vi "Digital Output Engine.vi"(5 "Main Engine Q":refnum<queue>, 7 "TCP Enigine Q":refnum<queue>, 8 "error in (no error)":errorcluster, 10 "Engine Name":string, 11 "Varient Data":variant) -> (0 "error out":errorcluster)   [LabVIEW 2024]
doc: "All Rights Reserved © 2017 SyncSols"
uses:
  Controls/Digital Output State Machine Data Cluster.ctl
  TCP Engine/Controls/TCP Engine I&O  Interupt Cluster.ctl
  Controls/DIO Configuration cluster.ctl
  Controls/DIO Interface Data.ctl
  SubVIs/Digital Dynamic Cluster.ctl
  Controls/DIO Commad Q Cluster.ctl
  Main Engine/Controls/Main Engine JSON Command State.ctl
  Host-DQMH/Configuration/DO Channel's.ctl
  Controls/Digital Output SMCases.ctl
  Main Engine/Controls/Main Engine Engine No.Options.ctl
  Host-DQMH/Configuration/All Interface Data.ctl
  Host-DQMH/Configuration/Analog Input Single Channel Data--Cluster.ctl
  Host-DQMH/Configuration/Config-Channel Type.ctl
  Host-DQMH/Configuration/Channel Sub-Type.ctl
  Analog Output/Controls/AO Timing Cluster.ctl
  Main Engine/Controls/Main Engine Config Confirmation Cluster.ctl
  <vilib>/DAQmx/create/channels.llb/DAQmx Create Channel (DO-Digital Output).vi
  TCP Engine/TCP Engine.lvlib
  Host-DQMH/Configuration/Configuration.lvlib
panel:
  out "Array":string[](array[string])
  in  "Data Cluster":T1={"Array"=[], "Boolean"=FALSE, "Engine Name"="", "Main Engine Response Q"=refnum, "TCP Engine Response Q"=refnum, "Varient Data"=variant(string ""), "Interupt Q"=refnum, "Start Notifier"=refnum, "Stop Notifier"=refnum, "DIO Configuration Cluster"={"Interface"="", "Interface Data"={"Command"="", "SubCmd"="", "Frequency"=0, "Data"=[]}}, "DO Task"="", "Command Q"=refnum, "DO Config Data"=[], "Log File Path"=path ""}
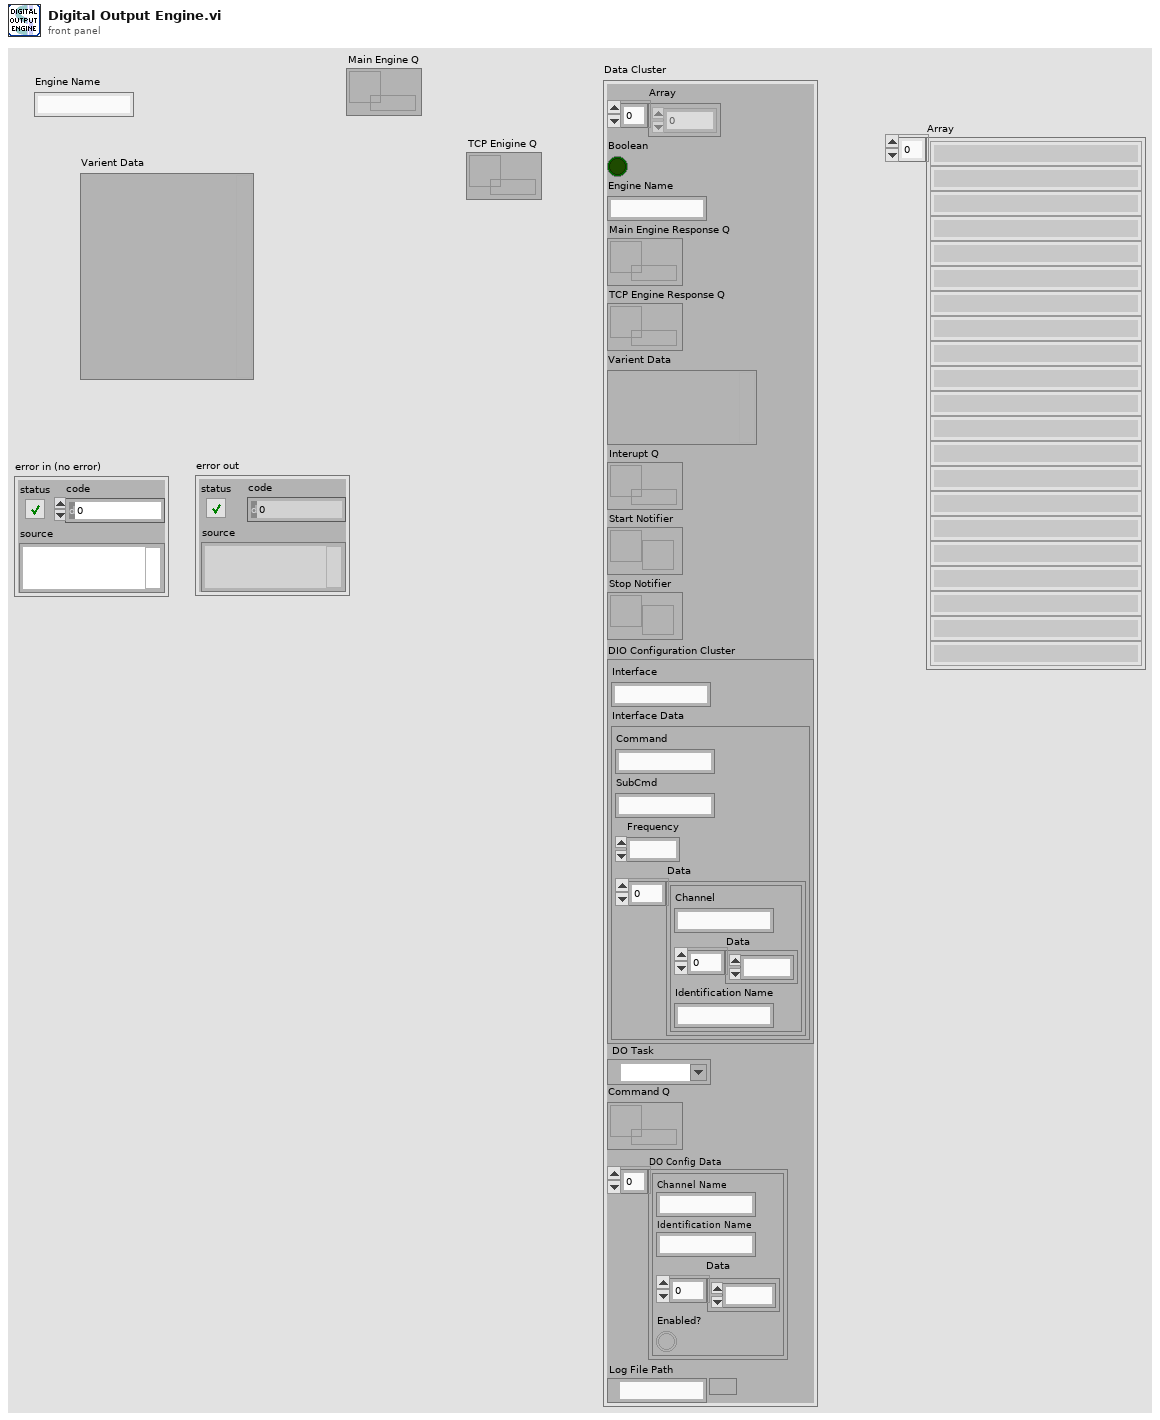
[diagram p1: front panel]
types:
  T1 = typedef "Digital Output State Machine Data Cluster.ctl" = cluster{"Array":dbl[], "Boolean":bool, "Engine Name":string, "Main Engine Response Q":refnum<queue>, "TCP Engine Response Q":refnum<queue>, "Varient Data":variant, "Interupt Q":refnum<queue>, "Start Notifier":refnum<notifier>, "Stop Notifier":refnum<notifier>, "DIO Configuration Cluster":T2, "DO Task":refnum<k21>, "Command Q":refnum<queue>, "DO Config Data":T5, "Log File Path":path}
  T2 = typedef "DIO Configuration cluster.ctl" = cluster{"Interface":string, "Interface Data":T3}
  T3 = typedef "DIO Interface Data.ctl" = cluster{"Command":string, "SubCmd":string, "Frequency":u16, "Data":T4[]}
  T4 = typedef "Digital Dynamic Cluster.ctl" = cluster{"Channel":string, "Data":u8[], "Identification Name":string}
  T5 = typedef "Configuration.lvlib/DO Channel's.ctl" = cluster{"Channel Name":string, "Identification Name":string, "Data":u8[], "Enabled?":bool}[]
  T6 = typedef "Digital Output SMCases.ctl" = enum16{">Poll", ".........State Machine.........", ">Init", ">Error", ">Exit", "..........Digital Output Engine Case..........", ">JSON to LVDATA", ">Gen Dyn Data", ">Get Command", ">Configure", ">Start", ">Generate", ">Stop"}
  T7 = typedef "DIO Commad Q Cluster.ctl" = cluster{"Interface":string, "Interface Data":cluster{"Command":string, "SubCmd":string, "Frequency":u16, "Data":T4[]}, "Command State":T8}
  T8 = typedef "Main Engine JSON Command State.ctl" = enum16{"Configure", "Start", "Exit"}
  T9 = typedef "TCP Engine.lvlib/TCP Engine I&O  Interupt Cluster.ctl" = cluster{" Stop":bool, "JSON Variant":variant}
  T10 = typedef "Main Engine Engine No.Options.ctl" = enum16{"Init", "Update", "Response", "Get"}
  T11 = typedef "Configuration.lvlib/All Interface Data.ctl" = cluster{"DI Config Data":T5, "DO Config Data":T5, "AI Config Data's":cluster{"Module Name":string, "AI Channel's Data":T12[], "Analog Input Timing":T15}[]}
  T12 = typedef "Configuration.lvlib/Analog Input Single Channel Data--Cluster.ctl" = cluster{"Channel Name":string, "Identification Name":string, "Channel Type":T13, "Sub-Type":T14, "Data":string, "Enabled?":bool}
  T13 = typedef "Configuration.lvlib/Config-Channel Type.ctl" = enum16{"Voltage", "Current", "Thermocouple", "Acclerometer"}
  T14 = typedef "Configuration.lvlib/Channel Sub-Type.ctl" = enum16{"None", "Pressure", "Force"}
  T15 = typedef "AO Timing Cluster.ctl" = cluster{"samples per channel":i32, "sample mode":i32, "Sampling Rate":dbl}
  T16 = typedef "Main Engine Config Confirmation Cluster.ctl" = cluster{"Command":string, "Interface":string, "Status":string, "Board":string}
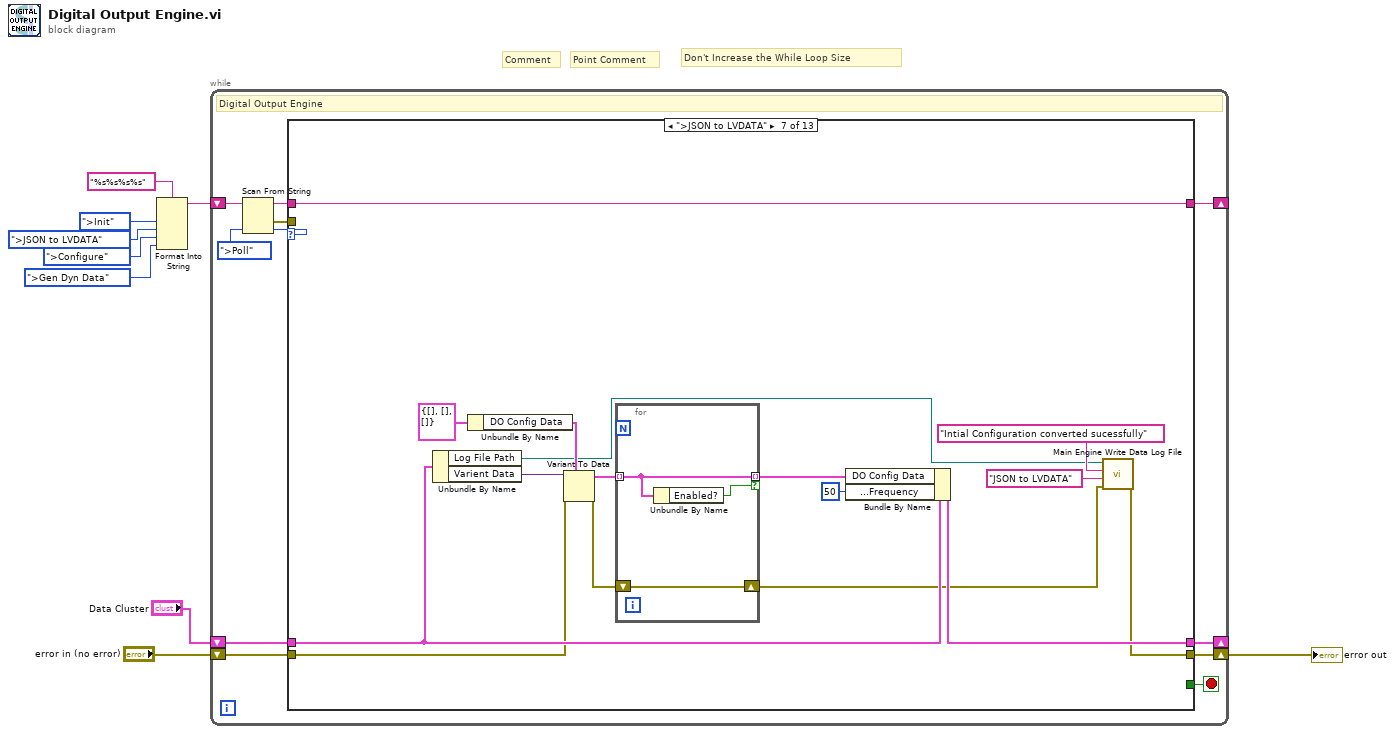
[diagram p0: block diagram]
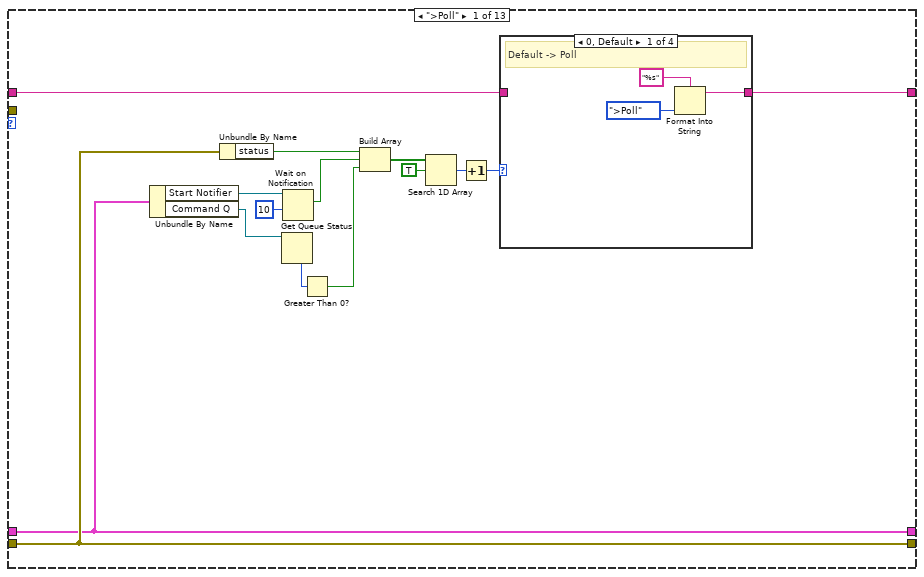
[diagram p2: hidden frame]
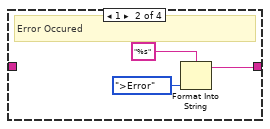
[diagram p3: hidden frame]
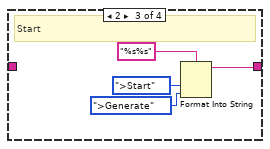
[diagram p4: hidden frame]
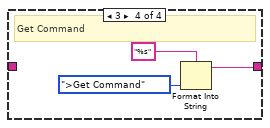
[diagram p5: hidden frame]
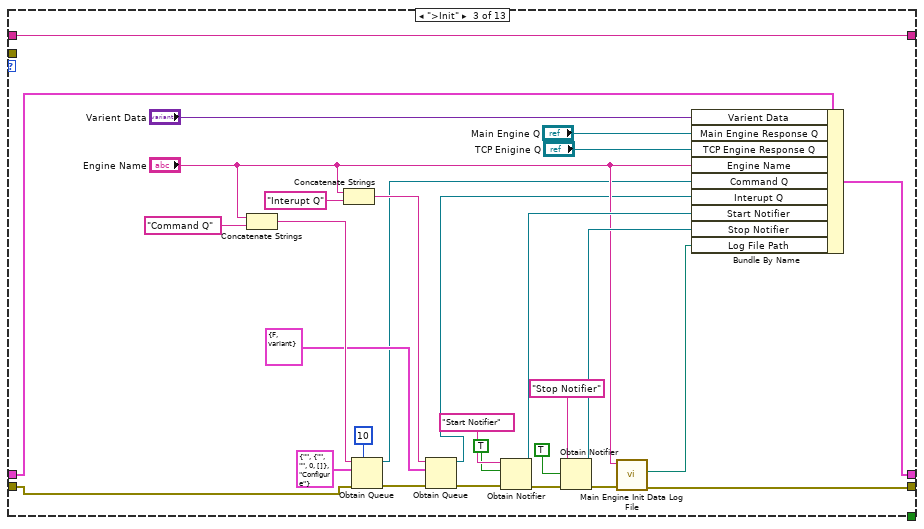
[diagram p7: hidden frame]
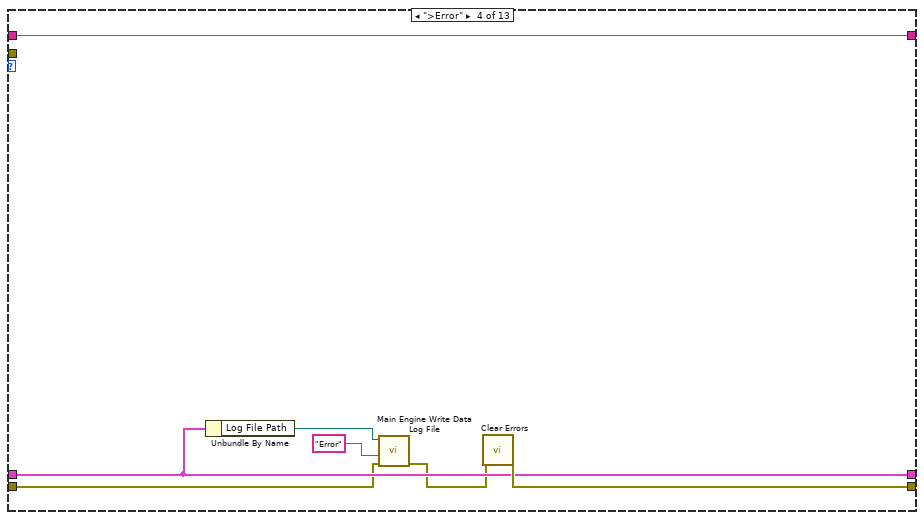
[diagram p8: hidden frame]
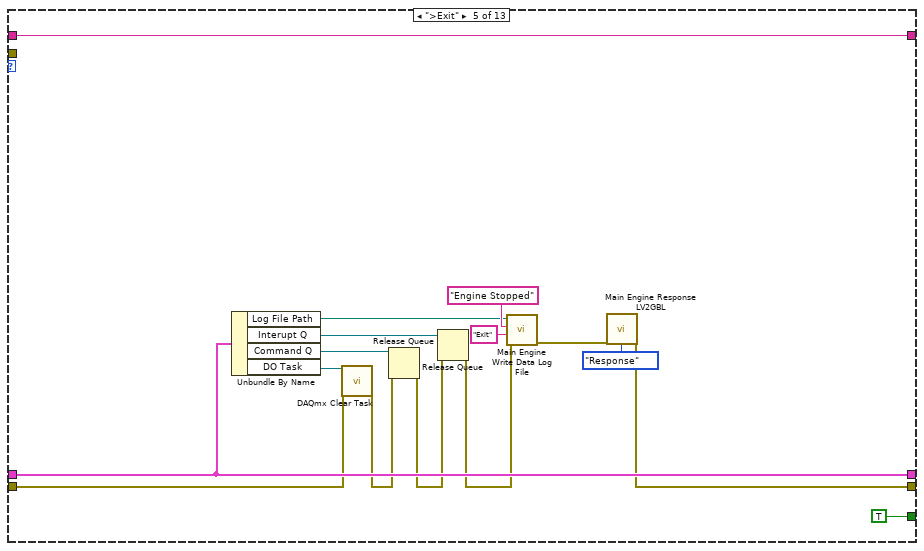
[diagram p9: hidden frame]
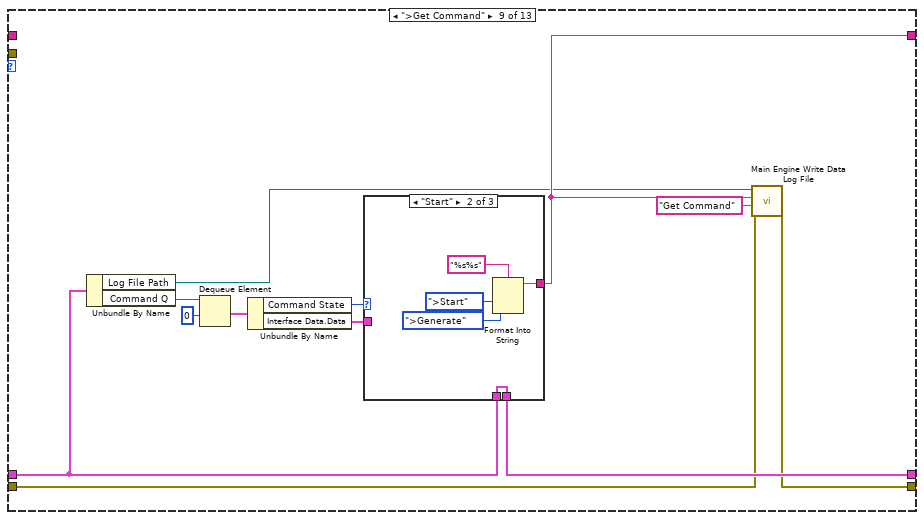
[diagram p12: hidden frame]
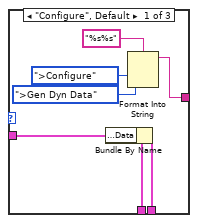
[diagram p13: hidden frame]
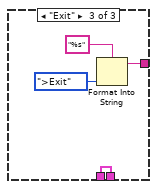
[diagram p14: hidden frame]
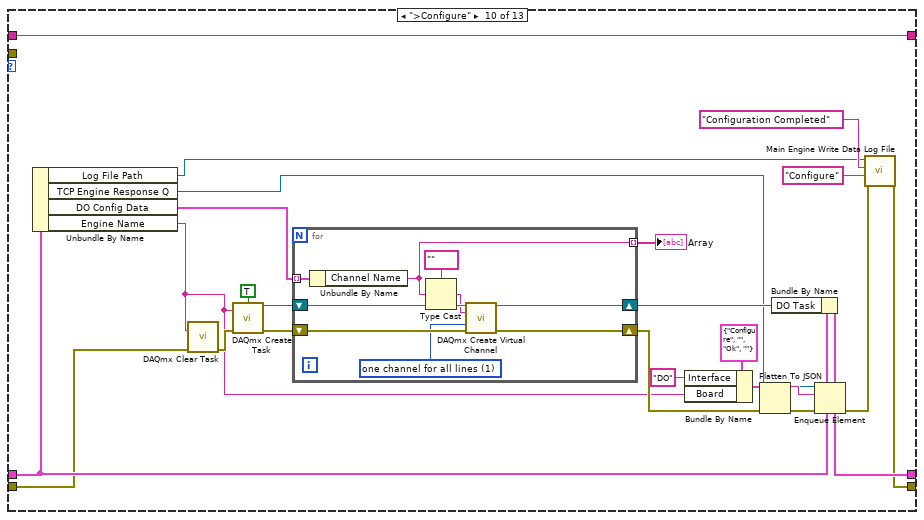
[diagram p15: hidden frame]
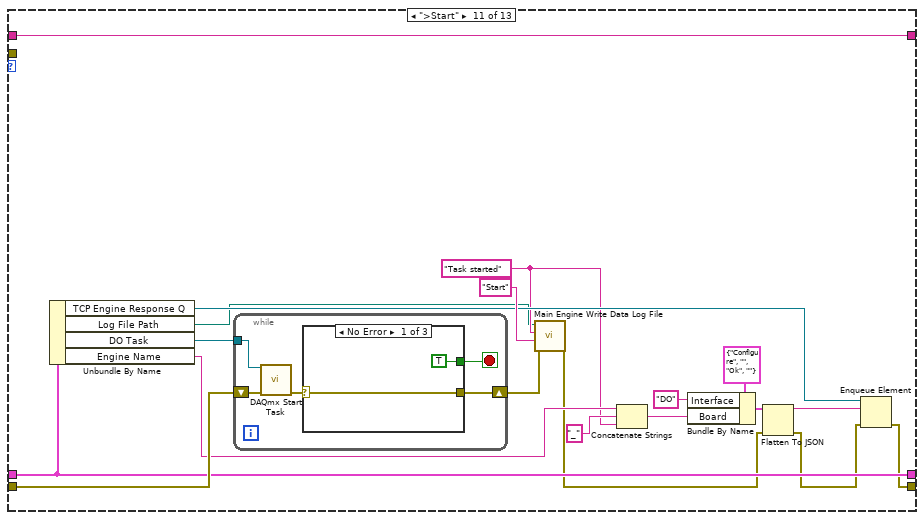
[diagram p16: hidden frame]
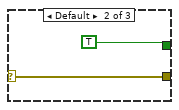
[diagram p17: hidden frame]
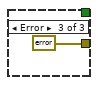
[diagram p18: hidden frame]
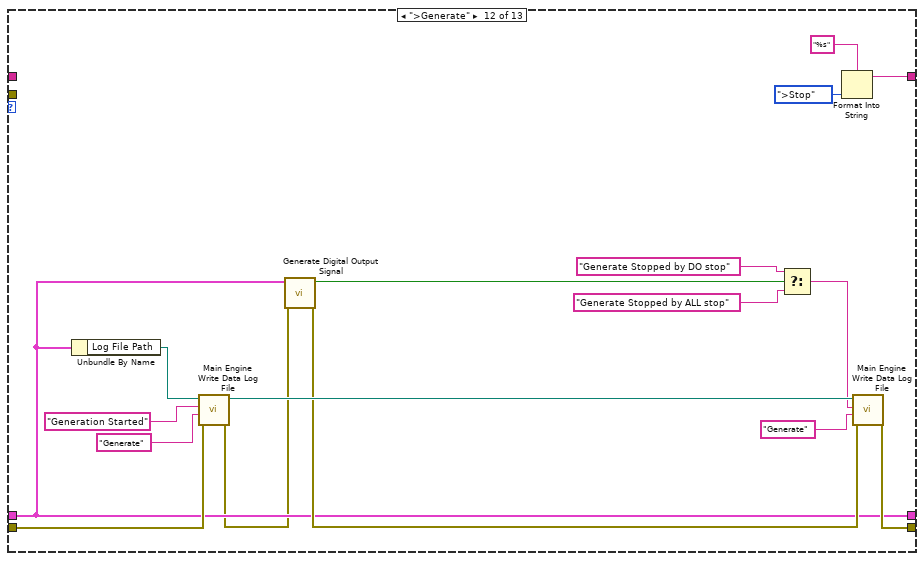
[diagram p19: hidden frame]
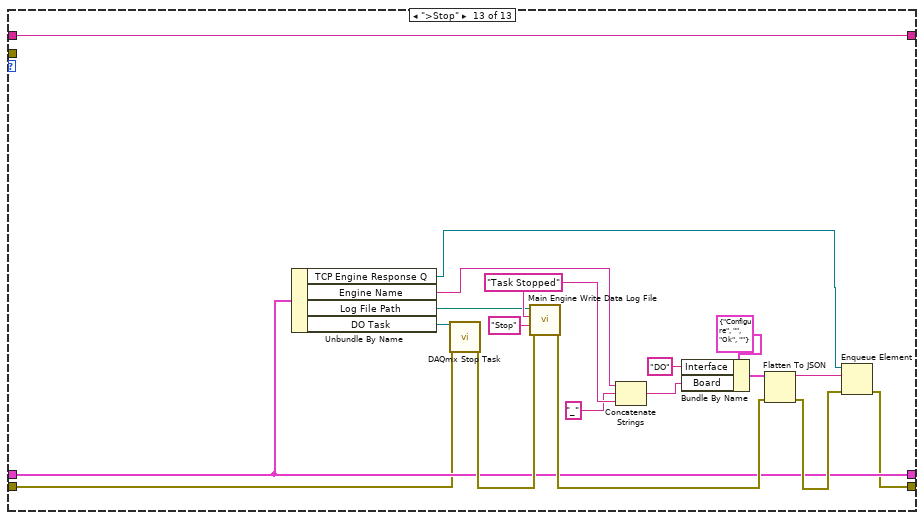
[diagram p20: hidden frame]
diagram:
  # "Don't Increase the While Loop Size"
  # "Point Comment"
  # "Comment"
  n1 = Format Into String(format string="%s%s%s%s", Digital_Output_SMCases.">Init" ("SM Cases Options"), Digital_Output_SMCases.">JSON to LVDATA" ("input 2"), Digital_Output_SMCases.">Configure" ("input 3"), Digital_Output_SMCases.">Gen Dyn Data" ("input 3")) -> (resulting string=w8:string)  [unwired: 2 in, 1 out]
  n2 = while {
    shift-right: [w15] -> _
    shift-left: w8 -> [w20]
    shift-right: [w13] -> w5
    shift-left: "error in (no error)" -> [w14]
    shift-right: [w11] -> _
    shift-left: "Data Cluster" -> [w10]
    stop <- w12 stop-if-true
    # "Digital Output Engine"
    n3 = Scan From String(input string=w20, default 1=Digital_Output_SMCases.">Poll" ("SM Cases Options")) -> (remaining string=w16:string, error out=w18:errorcluster, output 1=w17:T6)  [unwired: 3 in, 1 out]
    n4 = case shown="\">JSON to LVDATA\"" w17 {
      tunnel: w18 -> [_ _ _ _ _ _ _ _ _ _ _ _ _]
      tunnel: w16 -> [w35 w51 w80 w87 w103 w106 w122 w128 _ w180 w208 _ w254]
      tunnel: [w34 w51 w80 w87 w103 w106 w122 w128 w131 w180 w208 w229 w254] -> w15
      tunnel: w14 -> [w33 w50 w60 w83 w92 w105 w115 w126 w132 w176 w207 w235 w238]
      tunnel: [w33 w50 w61 w86 w90 w105 w119 w126 w133 w172 w191 w231 w237] -> w13
      tunnel: [_ _ _ _ TRUE _ _ _ _ _ _ _ _] -> w12
      tunnel: [w27 w49 w79 w84 w101 w104 w120 w127 w135 w174 w206 w221 w239] -> w11
      tunnel: w10 -> [w27 w49 w53 w84 w101 w104 w121 w127 w134 w179 w206 w221 w239]
      frame ">Poll" {
        n5 = Unbundle By Name(w27) -> ("Start Notifier"=w26:refnum<notifier>, "Command Q"=w24:refnum<queue>)
        n6 = Unbundle By Name(w33) -> ("status"=w32:bool)
        n7 = Get Queue Status(queue=w24) -> (# elements in queue=w23:i32)  [unwired: 2 in, 7 out]
        n8 = Wait on Notification(notifier=w26, timeout in ms (-1)=10) -> (notification=w25:bool)  [unwired: 2 in, 3 out]
        n9 = Greater Than 0?(x=w23) -> (x > 0?=w22:bool)
        n10 = Build Array(w32, w25, w22) -> (w31:bool[])
        n11 = Search 1D Array(1D array=w31, element=TRUE) -> (index of element=w29:i32)  [unwired: 1 in]
        n12 = Increment(x=w29) -> (x+1=w28:i32)
        n13 = case shown="0, Default" w28 {
          tunnel: w35 -> [_ _ _ _]
          tunnel: [w36 w39 w43 w46] -> w34
          frame 0, Default {
            # "Default -> Poll"
            n14 = Format Into String(format string="%s", Digital_Output_SMCases.">Poll" ("SM Cases Options")) -> (resulting string=w36:string)  [unwired: 2 in, 1 out]
          }
          frame 1 {
            # "Error Occured"
            n15 = Format Into String(format string="%s", Digital_Output_SMCases.">Error" ("SM Cases Options")) -> (resulting string=w39:string)  [unwired: 2 in, 1 out]
          }
          frame 2 {
            # "Start"
            n16 = Format Into String(format string="%s%s", Digital_Output_SMCases.">Start" ("SM Cases Options"), Digital_Output_SMCases.">Generate" ("input 2")) -> (resulting string=w43:string)  [unwired: 2 in, 1 out]
          }
          frame 3 {
            # "Get Command"
            n17 = Format Into String(format string="%s", Digital_Output_SMCases.">Get Command" ("SM Cases Options")) -> (resulting string=w46:string)  [unwired: 2 in, 1 out]
          }
        }
      }
      frame ".........State Machine........." {
      }
      frame ">Init" {
        n18 = Concatenate Strings("Engine Name", "Command Q" ("string")) -> (w76:string)
        n19 = Concatenate Strings("Engine Name", "Interupt Q" ("string")) -> (w73:string)
        n20 = Obtain Queue(max queue size (-1, unlimited)=10, name (unnamed)=w76, element data type=T7 {"Interface"="", "Interface Data"={"Command"="", "SubCmd"="", "Frequency"=0, "Data"=[]}, "Command State"=enum."Configure"} ("DIO Command Q Cluster"), error in (no error)=w60) -> (queue out=w58:refnum<queue>, error out=w78:errorcluster)  [unwired: 1 in, 1 out]
        n21 = Obtain Queue(name (unnamed)=w73, element data type=T9 {" Stop"=FALSE, "JSON Variant"=variant(string "")} ("I/O  Interupt Cluster"), error in (no error)=w78) -> (queue out=w56:refnum<queue>, error out=w66:errorcluster)  [unwired: 2 in, 1 out]
        n22 = Obtain Notifier(name (unnamed)="Start Notifier", notification data type=TRUE, error in (no error)=w66) -> (notifier out=w64:refnum<notifier>, error out=w71:errorcluster)  [unwired: 1 in, 1 out]
        n23 = Obtain Notifier(name (unnamed)="Stop Notifier", notification data type=TRUE, error in (no error)=w71) -> (notifier out=w63:refnum<notifier>, error out=w67:errorcluster)  [unwired: 1 in, 1 out]
        n24 = call "Main Engine Init Data Log File.vi"("error in"=w67, "Engine Name"="Engine Name") -> ("error out"=w61:errorcluster, "Log File Path"=w52:path)  [unwired: 8 in]
        n25 = Bundle By Name(cluster=w53, "Varient Data"="Varient Data", "Main Engine Response Q"="Main Engine Q", "TCP Engine Response Q"="TCP Enigine Q", "Engine Name"="Engine Name", "Command Q"=w58, "Interupt Q"=w56, "Start Notifier"=w64, "Stop Notifier"=w63, "Log File Path"=w52) -> (w79:T1)
      }
      frame ">Error" {
        n26 = Unbundle By Name(w84) -> ("Log File Path"=w81:path)
        n27 = call "Main Engine Write Data Log File.vi"("error in"=w83, "State"="Error" ("Input Data"), "Log file path In"=w81) -> ("error out"=w82:errorcluster)  [unwired: 7 in, 1 out]
        n28 = call <vilib>:"Clear Errors.vi"("error in (no error)"=w82) -> ("error out"=w86:errorcluster)  [unwired: 5 in, 1 out]
      }
      frame ">Exit" {
        n29 = Unbundle By Name(w101) -> ("Log File Path"=w88:path, "Interupt Q"=w99:refnum<queue>, "Command Q"=w100:refnum<queue>, "DO Task"=w91:refnum<k21>)
        n30 = call <vilib>:"DAQmx Clear Task.vi"("task in"=w91, "error in"=w92) -> ("error out"=w93:errorcluster)  [unwired: 13 in]
        n31 = Release Queue(queue=w100, error in (no error)=w93) -> (error out=w98:errorcluster)  [unwired: 1 in, 2 out]
        n32 = Release Queue(queue=w99, error in (no error)=w98) -> (error out=w97:errorcluster)  [unwired: 1 in, 2 out]
        n33 = call "Main Engine Write Data Log File.vi"("error in"=w97, "State"="Exit", "Input Data"="Engine Stopped", "Log file path In"=w88) -> ("error out"=w96:errorcluster)  [unwired: 6 in, 1 out]
        n34 = call "Main Engine Response LV2GBL.vi"("Options"=Main_Engine_Engine_No.Options."Response", "error in"=w96) -> ("error out"=w90:errorcluster)  [unwired: 7 in, 2 out]
      }
      frame "..........Digital Output Engine Case.........." {
      }
      frame ">JSON to LVDATA" {
        n35 = Unbundle By Name(w121) -> ("Log File Path"=w107:path, "Varient Data"=w116:variant)
        n36 = Unbundle By Name(T11 {"DI Config Data"=[], "DO Config Data"=[], "AI Config Data's"=[]} ("Interface Data")) -> ("DO Config Data"=w113:T5)
        n37 = Variant To Data(error in=w115, type=w113, Variant=w116) -> (data=w111:T5, error out=w109:errorcluster)
        n38 = for {
          tunnel: w111 -> [w125] mode=indexing
          tunnel: [w125] -> w110 mode=indexing if=w124
          shift-right: [w123] -> w108
          shift-left: w109 -> [w123]
          n39 = Unbundle By Name(w125) -> ("Enabled?"=w124:bool)
        }
        n40 = Bundle By Name(cluster=w121, "DO Config Data"=w110, "DIO Configuration Cluster.Interface Data.Frequency"=u16 50) -> (w120:T1)
        n41 = call "Main Engine Write Data Log File.vi"("error in"=w108, "State"="JSON to LVDATA", "Input Data"="Intial Configuration converted sucessfully", "Log file path In"=w107) -> ("error out"=w119:errorcluster)  [unwired: 6 in, 1 out]
      }
      frame ">Gen Dyn Data" {
      }
      frame ">Get Command" {
        n42 = Unbundle By Name(w134) -> ("Log File Path"=w129:path, "Command Q"=w140:refnum<queue>)
        n43 = Dequeue Element(queue=w140, timeout in ms (-1)=0) -> (element=w138:T7)  [unwired: 1 in, 3 out]
        n44 = Unbundle By Name(w138) -> ("Command State"=w137:T8, "Interface Data.Data"=w136:T4[])
        n45 = case shown="\"Start\"" w137 {
          tunnel: w134 -> [w147 w152 w156]
          tunnel: w136 -> [w146 _ _]
          tunnel: [w145 w152 w156] -> w135
          tunnel: [w142 w148 w153] -> w131
          frame "Configure", Default {
            n46 = Bundle By Name(cluster=w147, "DIO Configuration Cluster.Interface Data.Data"=w146) -> (w145:T1)
            n47 = Format Into String(format string="%s%s", Digital_Output_SMCases.">Configure" ("input 1"), Digital_Output_SMCases.">Gen Dyn Data" ("input 1")) -> (resulting string=w142:string)  [unwired: 2 in, 1 out]
          }
          frame "Start" {
            n48 = Format Into String(format string="%s%s", Digital_Output_SMCases.">Start" ("input 1"), Digital_Output_SMCases.">Generate" ("input 2")) -> (resulting string=w148:string)  [unwired: 2 in, 1 out]
          }
          frame "Exit" {
            n49 = Format Into String(format string="%s", Digital_Output_SMCases.">Exit" ("input 1")) -> (resulting string=w153:string)  [unwired: 2 in, 1 out]
          }
        }
        n50 = call "Main Engine Write Data Log File.vi"("error in"=w132, "State"="Get Command", "Input Data"=w131, "Log file path In"=w129) -> ("error out"=w133:errorcluster)  [unwired: 6 in, 1 out]
      }
      frame ">Configure" {
        n51 = Unbundle By Name(w179) -> ("Log File Path"=w157:path, "TCP Engine Response Q"=w165:refnum<queue>, "DO Config Data"=w159:T5, "Engine Name"=w161:string)
        n52 = call <vilib>:"DAQmx Clear Task.vi"("task in"=w161, "error in"=w176) -> ("error out"=w177:errorcluster)  [unwired: 13 in]
        n53 = call <vilib>:"DAQmx Create Task.vi"("new task name"=w161, "auto cleanup"=TRUE, "error in"=w177) -> ("task out"=w178:refnum<k21>, "error out"=w175:errorcluster)  [unwired: 11 in]
        n54 = for {
          tunnel: w159 -> [w185] mode=indexing
          shift-right: [w187] -> w173
          shift-left: w178 -> [w189]
          shift-right: [w186] -> w164
          shift-left: w175 -> [w188]
          tunnel: [w184] -> w158 mode=indexing
          w183 = 1 items=["one channel for each line", "one channel for all lines"] ("line grouping")
          n55 = Unbundle By Name(w185) -> ("Channel Name"=w184:string)
          n56 = Type Cast(type=tag "" ("lines"), x=w184) -> (*(type *) &x=w181:tag)
          n57 = call-poly <vilib>:"DAQmx Create Virtual Channel.vi"("task in"=w189, "lines"=w181, "line grouping"=w183, "error in"=w188) -> ("task out"=w187:refnum<k21>, "error out"=w186:errorcluster)  [unwired: 10 in]
        }
        "Array" <- w158
        n58 = Bundle By Name(cluster=T16 {"Command"="Configure", "Interface"="", "Status"="Ok", "Board"=""}, "Interface"="DO" ("SubCmd"), "Board"=w161) -> (w169:T16)
        n59 = Flatten To JSON(anything=w169, error in (no error)=w164) -> (JSON string=w168:string, 11:w162:errorcluster)  [unwired: 1 in]
        n60 = Bundle By Name(cluster=w179, "DO Task"=w173) -> (w174:T1)
        n61 = Enqueue Element(queue=w165, element=w168, error in (no error)=w162) -> (error out=w163:errorcluster)  [unwired: 1 in, 2 out]
        n62 = call "Main Engine Write Data Log File.vi"("error in"=w163, "State"="Configure", "Input Data"="Configuration Completed", "Log file path In"=w157) -> ("error out"=w172:errorcluster)  [unwired: 6 in, 1 out]
      }
      frame ">Start" {
        w195 = "Task started" ("Input Data")
        n63 = Unbundle By Name(w206) -> ("TCP Engine Response Q"=w198:refnum<queue>, "Log File Path"=w190:path, "DO Task"=w205:refnum<k21>, "Engine Name"=w196:string)
        n64 = while {
          tunnel: w205 -> [w212]
          shift-right: [w210] -> w203
          shift-left: w207 -> [w213]
          stop <- w209 stop-if-true
          n65 = call <vilib>:"DAQmx Start Task.vi"("task/channels in"=w212, "error in"=w213) -> ("error out"=w211:errorcluster)  [unwired: 12 in, 1 out]
          n66 = case shown="No Error" w211 {
            selector: w211 -> [w215 w217 _]
            tunnel: [w215 w217 errorcluster {"status"=FALSE, "code"=0, "source"=""} ("error IO")] -> w210
            tunnel: [TRUE TRUE _] -> w209
            frame No Error {
            }
            frame Default {
            }
            frame Error {
            }
          }
        }
        n67 = call "Main Engine Write Data Log File.vi"("error in"=w203, "State"="Start", "Input Data"=w195, "Log file path In"=w190) -> ("error out"=w193:errorcluster)  [unwired: 6 in, 1 out]
        n68 = Concatenate Strings(w196, "_", w195) -> (w194:string)
        n69 = Bundle By Name(cluster=T16 {"Command"="Configure", "Interface"="", "Status"="Ok", "Board"=""}, "Interface"="DO" ("SubCmd"), "Board"=w194) -> (w202:T16)
        n70 = Flatten To JSON(anything=w202, error in (no error)=w193) -> (JSON string=w201:string, 11:w192:errorcluster)  [unwired: 1 in]
        n71 = Enqueue Element(queue=w198, element=w201, error in (no error)=w192) -> (error out=w191:errorcluster)  [unwired: 1 in, 2 out]
      }
      frame ">Generate" {
        n72 = Unbundle By Name(w221) -> ("Log File Path"=w219:path)
        n73 = call "Main Engine Write Data Log File.vi"("error in"=w235, "State"="Generate", "Input Data"="Generation Started", "Log file path In"=w219) -> ("error out"=w220:errorcluster, "Log File Path Out"=w232:path)  [unwired: 6 in]
        n74 = call "Generate Digital Output Signal.vi"("error in"=w220, "Data Cluster"=w221) -> ("error out"=w226:errorcluster, "Generation Stop"=w225:bool)  [unwired: 8 in]
        n75 = Select(t="Generate Stopped by DO stop" ("State"), s=w225, f="Generate Stopped by ALL stop" ("State")) -> (s? t:f=w222:string)
        n76 = Format Into String(format string="%s", Digital_Output_SMCases.">Stop" ("input 1")) -> (resulting string=w229:string)  [unwired: 2 in, 1 out]
        n77 = call "Main Engine Write Data Log File.vi"("error in"=w226, "State"="Generate", "Input Data"=w222, "Log file path In"=w232) -> ("error out"=w231:errorcluster)  [unwired: 6 in, 1 out]
      }
      frame ">Stop" {
        w243 = "Task Stopped" ("Input Data")
        n78 = Unbundle By Name(w239) -> ("TCP Engine Response Q"=w250:refnum<queue>, "Engine Name"=w251:string, "Log File Path"=w236:path, "DO Task"=w245:refnum<k21>)
        n79 = call <vilib>:"DAQmx Stop Task.vi"("task/channels in"=w245, "error in"=w238) -> ("error out"=w246:errorcluster)  [unwired: 12 in, 1 out]
        n80 = call "Main Engine Write Data Log File.vi"("error in"=w246, "State"="Stop", "Input Data"=w243, "Log file path In"=w236) -> ("error out"=w252:errorcluster)  [unwired: 6 in, 1 out]
        n81 = Concatenate Strings(w251, "_", w243) -> (w248:string)
        n82 = Bundle By Name(cluster=T16 {"Command"="Configure", "Interface"="", "Status"="Ok", "Board"=""}, "Interface"="DO" ("SubCmd"), "Board"=w248) -> (w249:T16)
        n83 = Flatten To JSON(anything=w249, error in (no error)=w252) -> (JSON string=w247:string, 11:w253:errorcluster)  [unwired: 1 in]
        n84 = Enqueue Element(queue=w250, element=w247, error in (no error)=w253) -> (error out=w237:errorcluster)  [unwired: 1 in, 2 out]
      }
    }
  }
  "error out" <- w5
